vi "Logging Stopped.vi"(8 "error in (no error)":errorcluster, 11 "Logging in":refnum<class "Logging.lvclass">) -> (0 "error out":errorcluster, 3 "State Machine Actor out":refnum<class "State Machine Actor.lvclass">)   [LabVIEW 2024, in "Logging.lvlib" / "Logging.lvclass"]
uses:
  Logging.lvclass
  Logging.lvclass/Logging.ctl
  State Machine Actor/State Machine Actor/State Machine Actor.lvclass
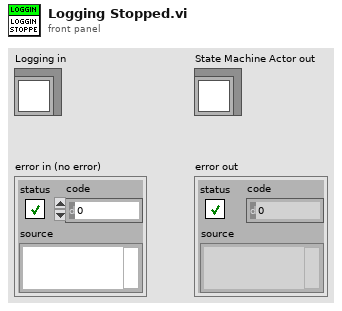
[diagram p1: front panel]
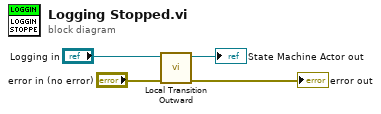
[diagram p0: block diagram]
diagram:
  n1 = call-dynamic "Local Transition Outward.vi"("error in (no error)"="error in (no error)", "State Machine Actor in"="Logging in") -> ("error out"=→"error out":errorcluster, "State Machine Actor out"=→"State Machine Actor out":refnum<class "State Machine Actor.lvclass">)  [unwired: 8 in]
